vi "DefineAcqSet.vi"(6 "Delay between send and receive [ms]":i32=100, 8 "error in (no error)":errorcluster, 10 "integration_time":T1, 11 "SCD in":refnum<class "SCD.lvclass">) -> (0 "error out":errorcluster, 3 "SCD out":refnum<class "SCD.lvclass">)   [LabVIEW 2023, in "horiba.lvlib" / "SCD.lvclass"]
doc: "Defines and sends the parameters for the acquisition set to perform the acquisition.\nIf the acquisition set is not defined, a single-point scan with default settings is performed.\nParameters that are not explicitly defined are set to their default values.\nParameters to define for the acquisition\n\nScan Count : Number of acquisitions to perform\nTime Steps : Time interval in seconds between acquisitions\nIntegration time: Time in Seconds\nExternal user defined parameter Returns an error if an acquisition is already in progress."
uses:
  SCD.lvclass
  acqSet.ctl
  b6349250-cb33-415b-847a-a7f5d99734f6.vi
  ca73f763-8e2b-4d84-8e4e-0e6044455bd1.vi
  <vilib>/JDP Science/JSONtext/Variant to JSON Text.vi
  <vilib>/JDP Science/JSONtext/Set Item.vi
  <vilib>/JDP Science/JSONtext/LVClass Serializer/JSONtext LVClass Serializer.lvclass
  SCD.lvclass/SCD.ctl
  GenericDevice/GenericDevice.lvclass
panel:
  # "Connector Pane"
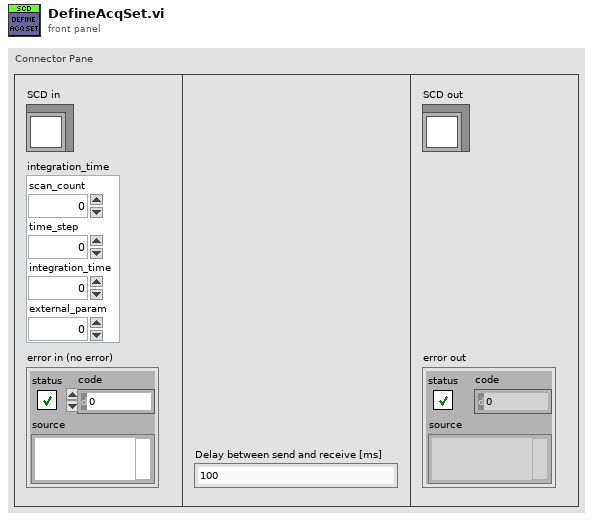
[diagram p1: front panel]
types:
  T1 = typedef "horiba.lvlib/SCD.lvclass/acqSet.ctl" = cluster{"scan_count":i32, "time_step":i32, "integration_time":i32, "external_param":i32}
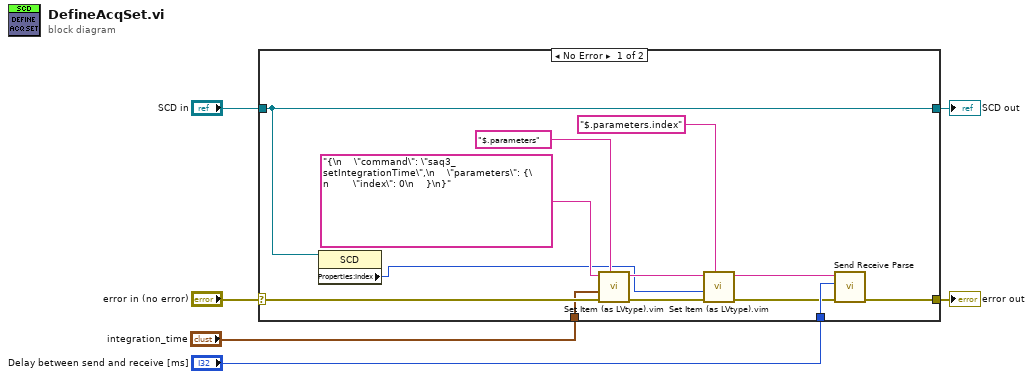
[diagram p0: block diagram]
diagram:
  n1 = case shown="No Error" "error in (no error)" {
    selector: "error in (no error)" -> [w17 w21]
    tunnel: [w15 w21] -> w2
    tunnel: [w18 w20] -> w4
    tunnel: "SCD in" -> [w18 w20]
    tunnel: "Delay between send and receive [ms]" -> [w14 _]
    tunnel: "integration_time" -> [w10 _]
    frame No Error {
      n2 = property class="SCD"(reference=w18) -> ("Properties:Index"=w7:i32)  [unwired: 1 in, 2 out]
      n3 = call "Set Item (as LVtype).vim"("$Path or Item Name"="$.parameters", "error in (no error)"=w17, "Anything"=w10, "JSON"="{\n    \"command\": \"saq3_setIntegrationTime\",\n    \"parameters\": {\n        \"index\": 0\n    }\n}") -> ("error out"=w16:errorcluster, "<JSON>"=w12:string)  [unwired: 4 in, 1 out]
      n4 = call "Set Item (as LVtype).vim"("$Path or Item Name"="$.parameters.index", "error in (no error)"=w16, "Anything"=w7, "JSON"=w12) -> ("error out"=w13:errorcluster, "<JSON>"=w11:string)  [unwired: 4 in, 1 out]
      n5 = call "Send Receive Parse.vi"("error in"=w13, "Delay between send and receive [ms]"=w14, "<JSON>"=w11) -> ("error out"=w15:errorcluster)  [unwired: 6 in, 2 out]
    }
    frame Error {
    }
  }
  "error out" <- w2
  "SCD out" <- w4
